vi "Find XML Descriptor.vi"(8 "error in":errorcluster, 11 "Project Path":path) -> (0 "error out":errorcluster, 2 "Found ?":bool, 3 "XML Path":path)   [LabVIEW 2019, in "Project XML Editor.lvclass"]
uses:
  Project XML Editor.lvclass
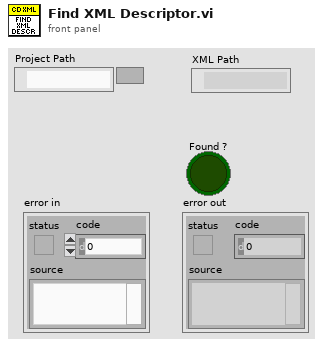
[diagram p1: front panel]
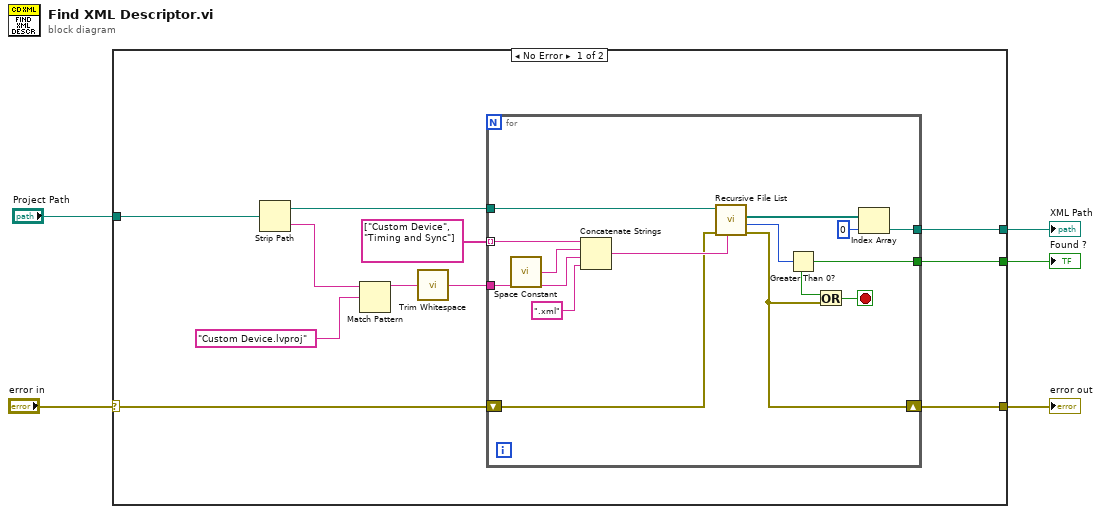
[diagram p0: block diagram]
diagram:
  n1 = case shown="No Error" "error in" {
    selector: "error in" -> [w8 w31]
    tunnel: "Project Path" -> [w10 _]
    tunnel: [w9 _] -> w4
    tunnel: [w7 w31] -> w2
    tunnel: [w6 _] -> w1
    frame No Error {
      n2 = Strip Path(path=w10) -> (stripped path=w13:path, name=w11:string)
      n3 = Match Pattern(string=w11, regular expression="Custom Device.lvproj") -> (before substring=w15:string)  [unwired: 1 in, 3 out]
      n4 = call <vilib>:"Trim Whitespace.vi"("string"=w15) -> ("trimmed string"=w16:string)  [unwired: 1 in]
      n5 = for {
        tunnel: w13 -> [w26]
        tunnel: string[] ["Custom Device", "Timing and Sync"] -> [w30] mode=indexing
        tunnel: w16 -> [w29]
        tunnel: [w20] -> w9
        tunnel: [w19] -> w6
        shift-right: [w17] -> w7
        shift-left: w8 -> [w18]
        stop <- w23 stop-if-true
        n6 = call <vilib>:"Space Constant.vi"() -> ("String"=w27:string)
        n7 = Concatenate Strings(w30, w27, w29, ".xml" ("string")) -> (w25:string)
        n8 = call <vilib>:"Recursive File List.vi"("pattern"=w25, "error in (no error)"=w18, "Folder Path"=w26) -> ("error out"=w17:errorcluster, "Number of Files"=w24:i32, "All Files in Dir"=w22:path[])  [unwired: 4 in, 2 out]
        n9 = Greater Than 0?(x=w24) -> (x > 0?=w19:bool)
        n10 = Or(x=w19, y=w17) -> (x .or. y?=w23:bool)
        n11 = Index Array(array=w22, index=0) -> (element=w20:path)
      }
    }
    frame Error {
    }
  }
  "XML Path" <- w4
  "error out" <- w2
  "Found ?" <- w1
